vi "Config Sample Rate.vi"(0 "VISA resource name":refnum<visa-resource-name>, 5 "Sample Rate (1: 0.25s)":u16(ring)=1 items=["0.1s", "0.25s", "0.5s", "1s", "2s", "5s"], 11 "error in (no error)":errorcluster) -> (4 "VISA resource name out":refnum<visa-resource-name>, 15 "error out":errorcluster)   [LabVIEW 2016, in "Yokogawa WT200 Series.lvlib"]
doc: "This VI sends the Display Update Rate Configuration commands to the WT210/WT230."
uses:
  Yokogawa WT200 Series.lvlib
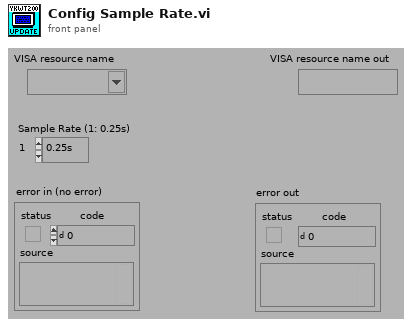
[diagram p1: front panel]
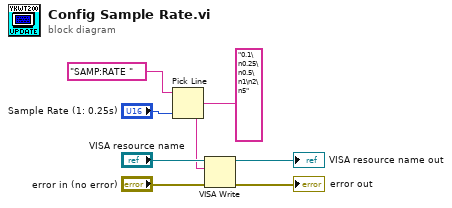
[diagram p0: block diagram]
diagram:
  n1 = Pick Line(string ("")="SAMP:RATE ", multi-line string="0.1\n0.25\n0.5\n1\n2\n5", line index="Sample Rate (1: 0.25s)") -> (output string=w1:string)
  n2 = VISA Write(VISA resource name="VISA resource name", write buffer=w1, error in (no error)="error in (no error)") -> (VISA resource name out=→"VISA resource name out":refnum<visa-resource-name>, error out=→"error out":errorcluster)  [unwired: 1 out]
